vi "Speed PI Control.vi"() -> ()   [LabVIEW 2016]
panel:
  in  "I-Gain":dbl(slide)=1.0 scale=0.0..2.0
  in  "P-Gain":dbl(slide)=1.0 scale=0.0..2.0
  in  "Setpoint Speed (rps)":dbl(slide) scale=-8.3..8.3
  out "Speed (rps)":dynamicdata(graph)
  in  "stop (F)":bool
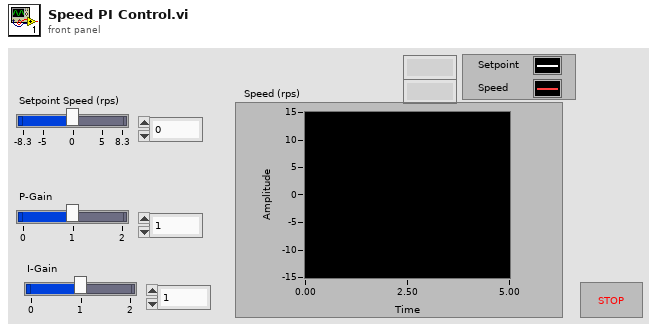
[diagram p1: front panel]
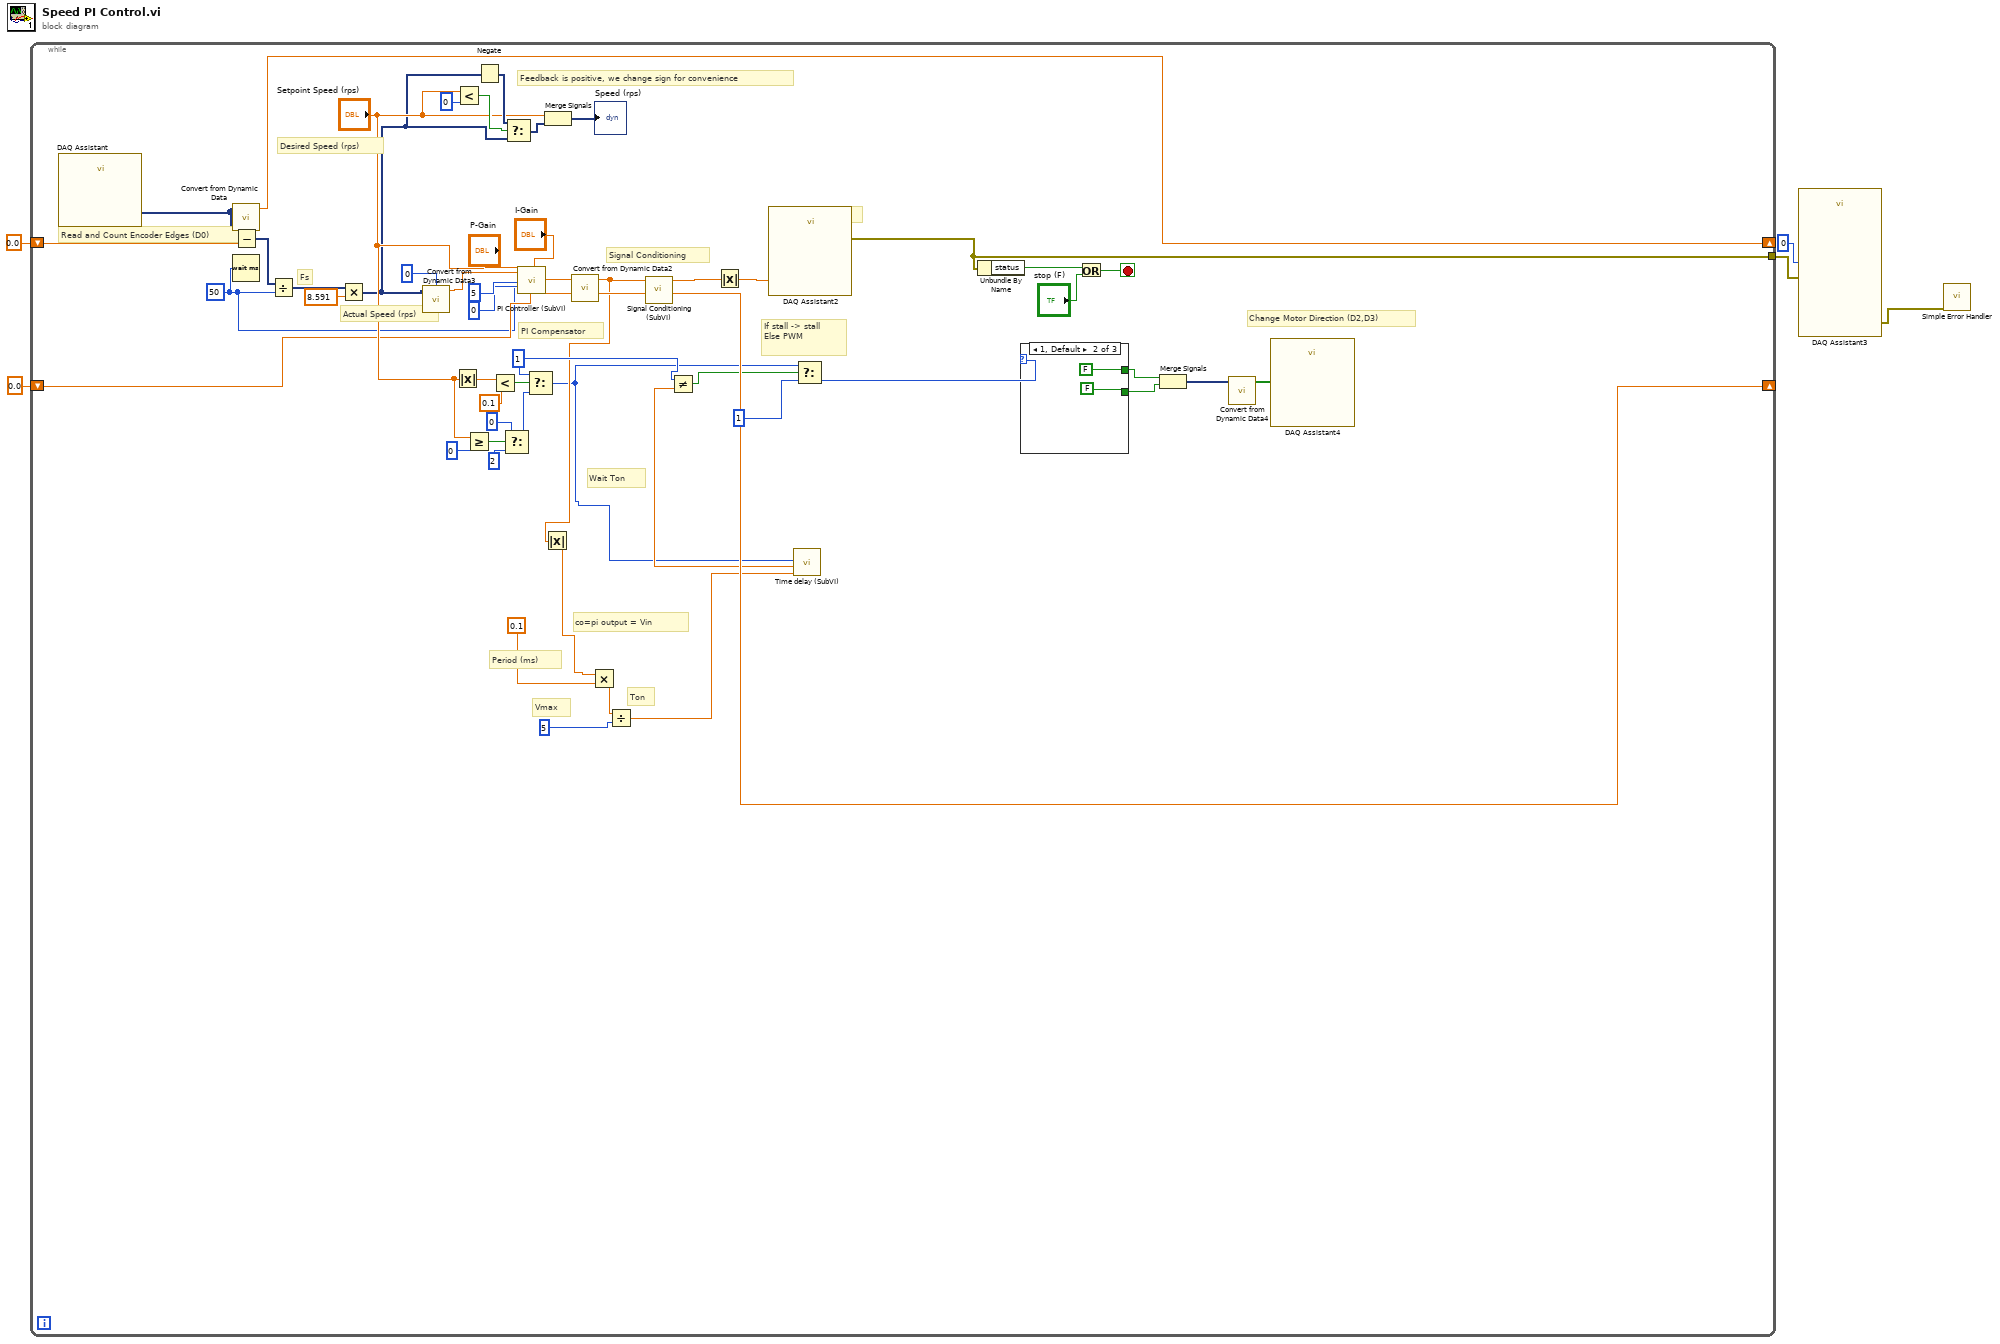
[diagram p0: block diagram]
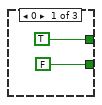
[diagram p2: hidden frame]
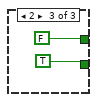
[diagram p3: hidden frame]
diagram:
  n1 = while {
    shift-right: [w58] -> _
    shift-left: 0.0 -> [w57]
    tunnel: [w53] -> w4
    shift-right: [w23] -> _
    shift-left: 0.0 -> [w26]
    stop <- w52 stop-if-true
    w16 = 1
    w25 = 50
    # "Change Motor Direction (D2,D3)"
    # "If stall -> stall\nElse PWM"
    # "Wait Ton"
    # "Ton"
    # "Vmax"
    # "co=pi output = Vin"
    # "Period (ms)"
    # "Desired Speed (rps)"
    # "Feedback is positive, we change sign for convenience"
    # "Signal Conditioning"
    # "PI Compensator"
    # "Fs"
    # "Actual Speed (rps)"
    # "Read and Count Encoder Edges (D0)"
    # "Plant Input (Ao0)"
    n2 = call "DAQ Assistant"() -> ("data"=w49:dynamicdata)  [unwired: 16 in, 3 out]
    n3 = call "Convert from Dynamic Data"("Dynamic Data Type"=w49) -> ("Scalar"=w58:dbl)  [unwired: 3 in]
    n4 = Wait (ms)(milliseconds to wait=w25) -> ()  [unwired: 1 out]
    n5 = Subtract(x=w49, y=w57) -> (x-y=w56:dynamicdata)
    n6 = Divide(x=w56, y=w25) -> (x/y=w55:dynamicdata)
    n7 = Multiply(x=w55, y=8.591) -> (x*y=w24:dynamicdata)
    n8 = call "Convert from Dynamic Data3"("Dynamic Data Type"=w24, "Channel"=0) -> ("Scalar"=w31:dbl)  [unwired: 2 in]
    n9 = Absolute Value(x="Setpoint Speed (rps)") -> (abs(x)=w43:dbl)
    n10 = Less?(x="Setpoint Speed (rps)", y=0) -> (x < y?=w34:bool)
    n11 = Greater Or Equal?(x="Setpoint Speed (rps)", y=0) -> (x >= y?=w46:bool)
    n12 = Negate(x=w24) -> (-x=w33:dynamicdata)
    n13 = Less?(x=w43, y=0.1) -> (x < y?=w41:bool)
    n14 = Select(t=0, s=w46, f=2) -> (s? t:f=w40:i32)
    n15 = Select(t=w33, s=w34, f=w24) -> (s? t:f=w35:dynamicdata)
    n16 = call "PI Controller (SubVI).vi"("sp"="Setpoint Speed (rps)", "pv"=w31, "maxim"=5, "minim"=0, "p"="P-Gain", "errsum"=w26, "i"="I-Gain", "h"=w25) -> ("output variable"=w22:dbl, "errsum"=w23:dbl)  [unwired: 18 in]
    n17 = Select(t=w16, s=w41, f=w40) -> (s? t:f=w11:i32)
    n18 = Merge Signals("Setpoint Speed (rps)", w35) -> (→"Speed (rps)":dynamicdata)
    n19 = call "Convert from Dynamic Data2"("Dynamic Data Type"=w22) -> ("Scalar"=w13:dbl)  [unwired: 3 in]
    n20 = Absolute Value(x=w13) -> (abs(x)=w12:dbl)
    n21 = Multiply(x=w12, y=0.1) -> (x*y=w21:dbl)
    n22 = Divide(x=w21, y=5) -> (x/y=w18:dbl)
    n23 = call "Signal Conditioning (SubVI).vi"("Input"=w13) -> ("Output"=w38:dbl)  [unwired: 10 in]
    n24 = Absolute Value(x=w38) -> (abs(x)=w39:dbl)
    n25 = call "DAQ Assistant2"("data"=w39) -> ("error out"=w53:errorcluster)  [unwired: 17 in, 1 out]
    n26 = call "Time delay (SubVI).vi"(6:w18, "input"=w11) -> ("Output"=w15:dbl)  [unwired: 7 in]
    n27 = Not Equal?(x=w16, y=w15) -> (x != y?=w17:bool)
    n28 = Select(t=w11, s=w17, f=1) -> (s? t:f=w6:i32)
    n29 = Unbundle By Name(w53) -> ("status"=w50:bool)
    n30 = case shown="1, Default" w6 {
      tunnel: [TRUE FALSE FALSE] -> w8
      tunnel: [FALSE FALSE TRUE] -> w7
      frame 0 {
      }
      frame 1, Default {
      }
      frame 2 {
      }
    }
    n31 = Or(x=w50, y="stop (F)") -> (x .or. y?=w52:bool)
    n32 = Merge Signals(w8, w7) -> (w10:dynamicdata)
    n33 = call "Convert from Dynamic Data4"("Dynamic Data Type"=w10) -> ("Array"=w9:bool[])  [unwired: 3 in]
    n34 = call "DAQ Assistant4"("data"=w9) -> ()  [unwired: 17 in, 2 out]
  }
  n35 = call "DAQ Assistant3"("data"=0, "error in"=w4) -> ("error out"=w2:errorcluster)  [unwired: 16 in, 1 out]
  n36 = call <vilib>:"Simple Error Handler.vi"("error in (no error)"=w2) -> ()  [unwired: 4 in, 5 out]
